vi "Build Spec Engine.vi"(9 "Action":T1) -> (1 "Output":string)   [LabVIEW 2019, in "NIVS_Consolidated_CDW_MetaDataObj.lvclass"]
doc: "Constants, which are necessary for the <B>CD Engine LLB</B> in the generated custom device."
uses:
  NIVS_Consolidated_CDW_MetaDataObj.lvclass
  Build Spec Engine.ctl
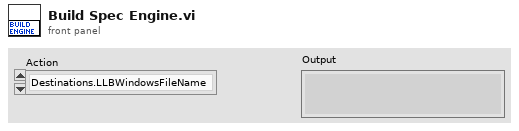
[diagram p1: front panel]
types:
  T1 = typedef "NIVS_Consolidated_CDW_MetaDataObj.lvclass/Build Spec Engine.ctl" = enum16{"Destinations.LLBWindowsFileName", "Destinations.LLBVxWorksFileName", "Destinations.LLBPharlapFileName", "Destinations.LLBLinuxARMFileName", "Destinations.LLBLinux64FileName", "Destinations.PPLWindowsFileName", "Destinations.PPLLinux64FileName"}
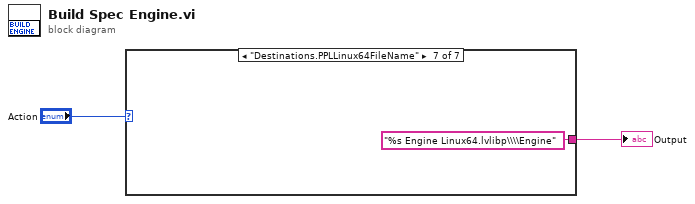
[diagram p0: block diagram]
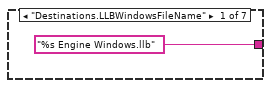
[diagram p2: hidden frame]
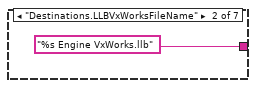
[diagram p3: hidden frame]
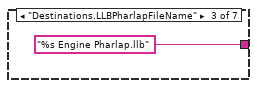
[diagram p4: hidden frame]
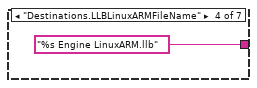
[diagram p5: hidden frame]
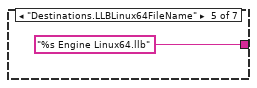
[diagram p6: hidden frame]
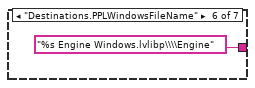
[diagram p7: hidden frame]
diagram:
  n1 = case shown="\"Destinations.PPLLinux64FileName\"" "Action" {
    tunnel: ["%s Engine Windows.llb" "%s Engine VxWorks.llb" "%s Engine Pharlap.llb" "%s Engine LinuxARM.llb" "%s Engine Linux64.llb" "%s Engine Windows.lvlibp\\\\Engine" "%s Engine Linux64.lvlibp\\\\Engine"] -> w2
    frame "Destinations.LLBWindowsFileName" {
    }
    frame "Destinations.LLBVxWorksFileName" {
    }
    frame "Destinations.LLBPharlapFileName" {
    }
    frame "Destinations.LLBLinuxARMFileName" {
    }
    frame "Destinations.LLBLinux64FileName" {
    }
    frame "Destinations.PPLWindowsFileName" {
    }
    frame "Destinations.PPLLinux64FileName" {
    }
  }
  "Output" <- w2
